vi "DC motor Circuit.vi"() -> ()   [LabVIEW 2014]
uses:
  <vilib>/Simulation/Scripting/Companion Diagram/SimConfigNode/SimParams.ctl
  <vilib>/Simulation/Scripting/Companion Diagram/SimConfigNode/_simSolvers.ctl
  <vilib>/Simulation/Implementation/Shared/SIMSCR Execution Mode.ctl
  <vilib>/Simulation/Param Hierarchy/Typedefs/SIMPH Param Control Actions.ctl
  <vilib>/Simulation/Implementation/Shared/SIM limit type.ctl
  <vilib>/Simulation/Implementation/Shared/NILVSim_ParamChanged.vi
  <vilib>/Simulation/Implementation/Shared/NILVSIM_BeginStep.vi
  <vilib>/Simulation/DataSources/Implementation/NILVSim Step.llb/SIM Step (scalar).vi
  <vilib>/Simulation/ContinuousLinear/Implementation/NILVSim Integrator new.llb/SIM Integrator distributor (scalar).vi
  <vilib>/Simulation/SignalArithmetic/Implementation/NILVSim Gain.llb/SIM Gain (scalar).vi
  <vilib>/Simulation/SignalDisplay/Implementation/NILVSim Time Waveform.llb/SIM Time Waveform (vector).vi
  <vilib>/Simulation/ContinuousLinear/Implementation/NILVSim Integrator new.llb/SIM Integrator collector (scalar).vi
  <vilib>/Simulation/Implementation/Shared/NILVSim_Manager.vi
  <vilib>/Utility/error.llb/Clear Errors.vi
  <vilib>/Simulation/Implementation/Shared/NILVSim_FinalizeModel.vi
  <vilib>/Simulation/Implementation/Shared/SIM Unbundle Sim Info.vi
  <vilib>/Simulation/Implementation/Shared/NILVSim_Initialize.vi
  <vilib>/Simulation/Utility/Implementation/NILVSim Get Time and IsAcceptedStep.vi
  <vilib>/Simulation/Implementation/Shared/SIMSH Read Queue.vi
  <vilib>/Simulation/Implementation/Shared/NILVSim_GetModelError.vi
  <vilib>/Simulation/Implementation/Shared/SIM Bundle Sim Info.vi
  <vilib>/Simulation/Scripting/Companion Diagram/SimConfigNode/SimDog.xnode
  <vilib>/Simulation/Implementation/XNodeFramework/SimXNode/SimX.xnode
  <vilib>/Simulation/ContinuousLinear/Implementation/NILVSim Integrator new.llb/SIM Integrator (scalar).vi
  <vilib>/Simulation/Implementation/Shared/NI_SIM_Implementation.lvlib
panel:
  in  "Km":dbl=3.5
  in  "Rm":dbl=1.0
  in  "Jm":dbl=0.1
  in  "Ke":dbl=3.5
  in  "L":dbl=0.1
  in  "R":dbl=3.0
  in  "Final time":dbl=15.0
  out "Waveform Chart 2":waveform(dbl)[](graph)=[{"t0"=timestamp(10 s since 1904-01-01), "dt"=1.0, "Y"=[1.0]}, {"t0"=timestamp(10 s since 1904-01-01), "dt"=1.0, "Y"=[0.49989915247330113]}]
  # "Title: DC motor Circuit, Bond Graph\nAuthor: Jad Saud \nDate: 2019.09.19\nVersion: v1.0"
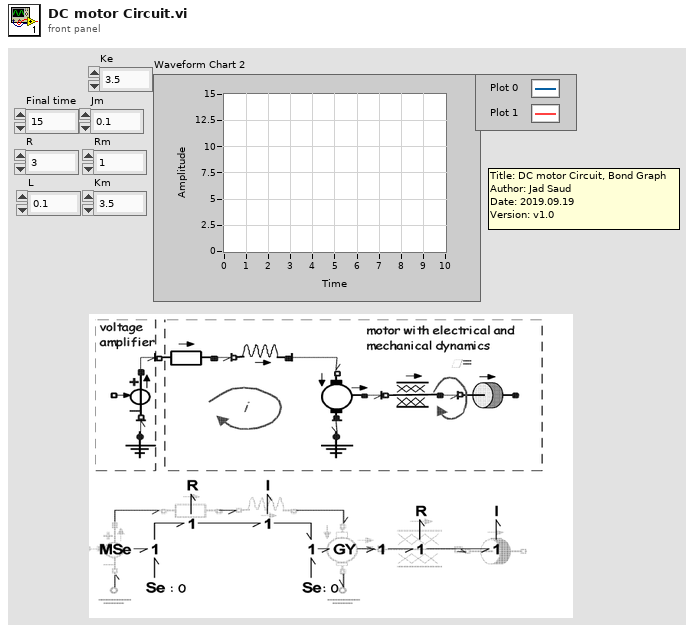
[diagram p1: front panel]
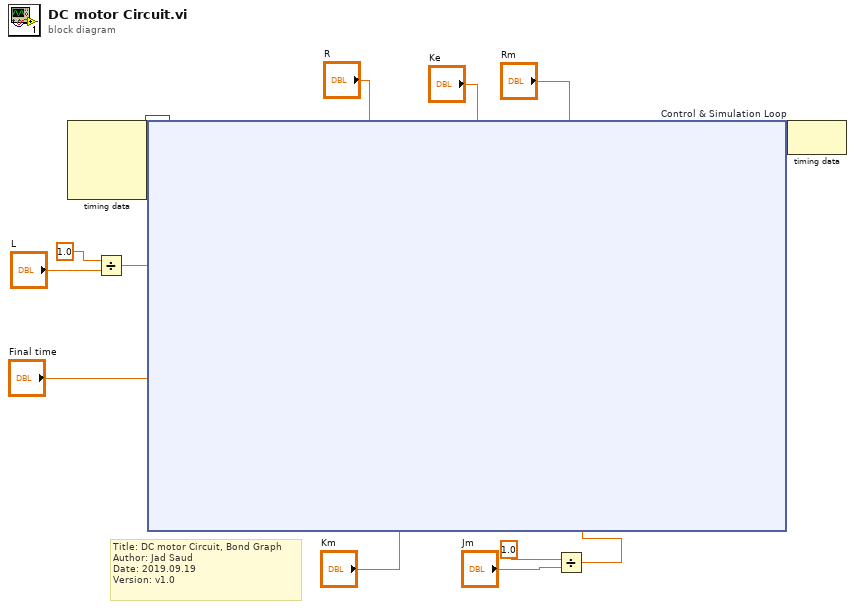
[diagram p0: block diagram]
diagram:
  # "Title: DC motor Circuit, Bond Graph\nAuthor: Jad Saud \nDate: 2019.09.19\nVersion: v1.0"
  n1 = node-c288() -> (w13:variant)  [unwired: 4 in]
  n2 = Divide(x=1.0, y="L") -> (x/y=w4:dbl)
  n3 = Divide(x=1.0, y="Jm") -> (x/y=w1:dbl)
  n4 = node-c254 "Control & Simulation Loop"(w13, "Final time", "R", w4, "Ke", w1, "Rm", "Km") -> (w12:variant)
  n5 = node-c288(w12) -> ()  [unwired: 1 out]
